vi "_initData.vi"(8 "error in (no error)":errorcluster, 10 "name":string) -> (0 "error out":errorcluster, 3 "DB Ref(dup)":T1)   [LabVIEW 2014, in "TagDB(dev).lvlib"]
doc: "初始化内部数据引用"
uses:
  TagDB(dev).lvlib
  tagDB_Def.ctl
  _DEF-DATA.ctl
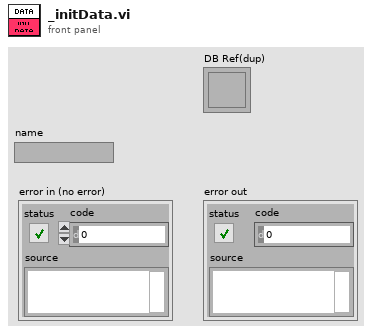
[diagram p1: front panel]
types:
  T1 = typedef "TagDB(dev).lvlib/tagDB_Def.ctl" = refnum<k1>
  T2 = typedef "TagDB(dev).lvlib/_DEF-DATA.ctl" = cluster{"data hashmap":variant, "DataChangeFlag":i64, "ItemChangeFlag":i64, "name":string, "Tag Adding Lock?":bool}
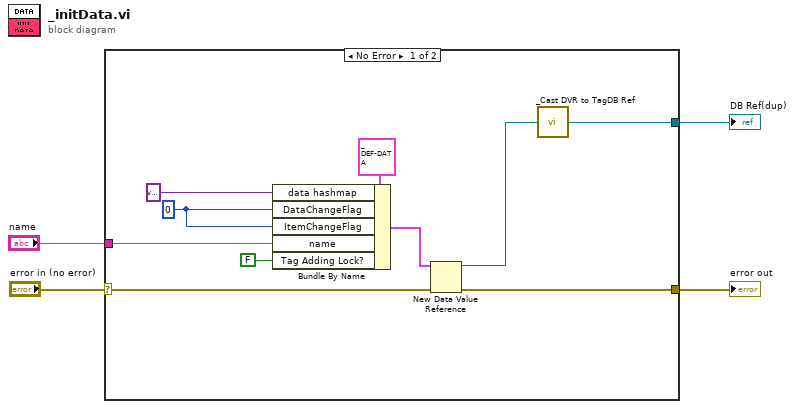
[diagram p0: block diagram]
diagram:
  n1 = case shown="No Error" "error in (no error)" {
    selector: "error in (no error)" -> [w13 w15]
    tunnel: [w14 _] -> w4
    tunnel: [w12 w15] -> w3
    tunnel: "name" -> [w6 _]
    frame No Error {
      w7 = i64 0 ("DataChangeFlag")
      n2 = Bundle By Name(cluster=T2 {"data hashmap"=variant, "DataChangeFlag"=0, "ItemChangeFlag"=0, "name"="", "Tag Adding Lock?"=FALSE} ("data def"), "data hashmap"=variant ("msg hashmap"), "DataChangeFlag"=w7, "ItemChangeFlag"=w7, "name"=w6, "Tag Adding Lock?"=FALSE) -> (w10:T2)
      n3 = New Data Value Reference(data value=w10, error in=w13) -> (data value reference=w9:refnum<data-value>, error out=w12:errorcluster)
      n4 = call "_Cast DVR to TagDB Ref.vi"("DVR"=w9) -> ("TagDB"=w14:T1)  [unwired: 4 in]
    }
    frame Error {
    }
  }
  "DB Ref(dup)" <- w4
  "error out" <- w3
